vi "PMX_SendCommand.vi"(8 "Error in":errorcluster, 10 "Command":string="idn?", 11 "Device":refnum<k24>) -> (0 "Error out":errorcluster, 2 "Answer":string, 3 "Device":refnum<k24>)   [LabVIEW 2016]
doc: "Sends a command to the device and returns its answer.\n\nCommand: Command to send to the device (see manual of the device for details)\nAnswer: Answer of the device according to sent command"
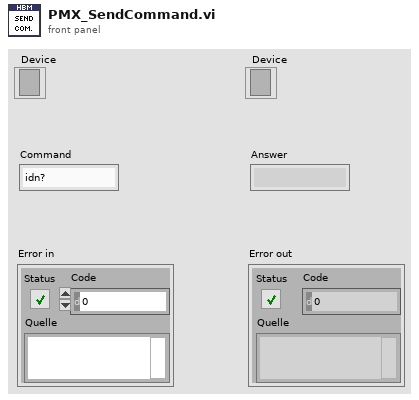
[diagram p1: front panel]
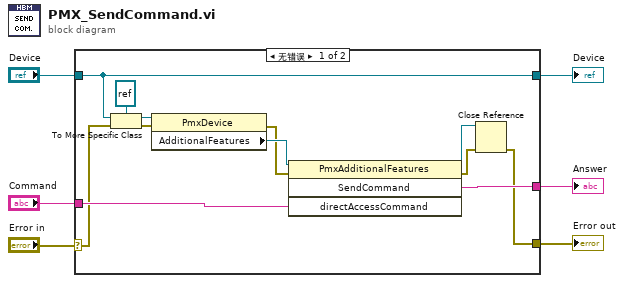
[diagram p0: block diagram]
diagram:
  n1 = case shown="无错误" "Error in" {
    selector: "Error in" -> [w11 w20]
    tunnel: "Device" -> [w12 w19]
    tunnel: [w12 w19] -> w5
    tunnel: [w7 w20] -> w3
    tunnel: [w14 _] -> w2
    tunnel: "Command" -> [w13 _]
    frame No Error {
      n2 = To More Specific Class(target class=refnum<k24> refnum ("Zielklasse"), reference=w12, error in=w11) -> (specific class reference=w18:refnum<k24>, error out=w15:errorcluster)
      n3 = property on="Eigenschaftsknoten" class="PmxDevice"(reference=w18, error in=w15) -> (error out=w16:errorcluster, "AdditionalFeatures"=w17:refnum<k24>)  [unwired: 1 out]
      n4 = invoke on="Methodenknoten" class="PmxAdditionalFeatures" method="SendCommand"(reference=w17, error in=w16, "directAccessCommand"=w13) -> (reference out=w8:refnum<k24>, error out=w9:errorcluster, "SendCommand"=w14:string)  [unwired: 1 in, 1 out]
      n5 = Close Reference(reference=w8, error in (no error)=w9) -> (error out=w7:errorcluster)
    }
    frame Error {
    }
  }
  "Error out" <- w3
  "Device" <- w5
  "Answer" <- w2
